vi "prueba1_520.vi"() -> ()   [LabVIEW 2011]
panel:
  out "Temperatura Mayor":dbl
  out "61-100":bool
  out "31-60":bool
  out "1-30":bool
  out "temperaturaProm":dbl
  out "temperatura":i32(slide) scale=0.0..100.0
  # "Generar la temperatura entre 1-100\nel programa se detiene cuando la\ntemperatura es mayor a 90.\nAl final debera de presentar la\ntemperatura promedio.\nDurante el programa se ejecute\ndebera de encender los led de acuerdo\nal rango.\nobtener la temperatura mayor"
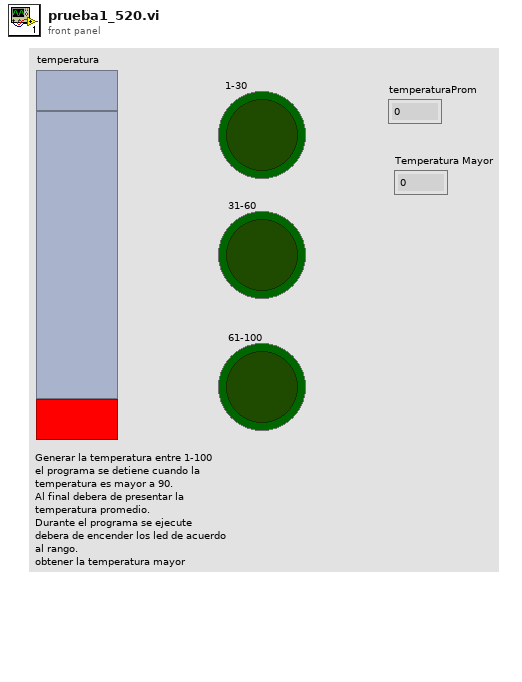
[diagram p1: front panel]
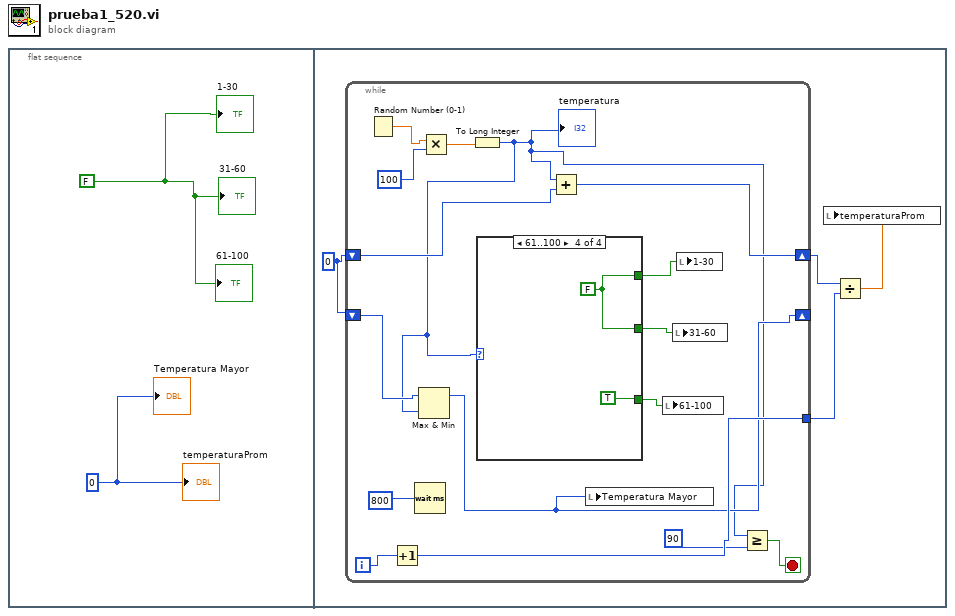
[diagram p0: block diagram]
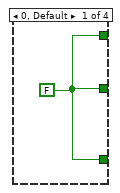
[diagram p2: hidden frame]
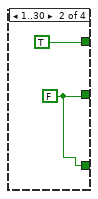
[diagram p3: hidden frame]
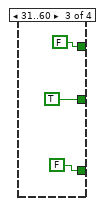
[diagram p4: hidden frame]
diagram:
  n1 = flat-sequence {
    frame #0 {
      w2 = FALSE
      w1 = 0
      "temperaturaProm" <- w1
      "1-30" <- w2
      "31-60" <- w2
      "61-100" <- w2
      "Temperatura Mayor" <- w1
    }
    frame #1 {
      w3 = 0
      n2 = while {
        shift-right: [w15] -> w6
        shift-left: w3 -> [w18]
        shift-right: [w10] -> _
        shift-left: w3 -> [w11]
        tunnel: [w16] -> w5
        i -> [w17]
        stop <- w9 stop-if-true
        n3 = Random Number (0-1)() -> (number: 0 to 1=w19:dbl)
        n4 = Increment(x=w17) -> (x+1=w16:i32)
        n5 = Wait (ms)(milliseconds to wait=800) -> ()  [unwired: 1 out]
        n6 = Multiply(x=w19, y=100) -> (x*y=w21:dbl)
        n7 = To Long Integer(number=w21) -> (32bit integer=w7:i32)
        "temperatura" <- w7
        n8 = Max & Min(x=w11, y=w7) -> (max(x,y)=w10:i32)  [unwired: 1 out]
        n9 = case shown="61..100" w7 {
          tunnel: [w23 TRUE FALSE w29] -> w14
          tunnel: [w23 w24 FALSE TRUE] -> w13
          tunnel: [w23 w24 TRUE w29] -> w12
          frame 0, Default {
            w23 = FALSE
          }
          frame 1..30 {
            w24 = FALSE
          }
          frame 31..60 {
          }
          frame 61..100 {
            w29 = FALSE
          }
        }
        n10 = Add(x=w7, y=w18) -> (x+y=w15:i32)
        n11 = local write "Temperatura Mayor"(w10) -> ()
        n12 = local write "61-100"(w13) -> ()
        n13 = local write "31-60"(w12) -> ()
        n14 = local write "1-30"(w14) -> ()
        n15 = Greater Or Equal?(x=w7, y=90) -> (x >= y?=w9:bool)
      }
      n16 = Divide(x=w6, y=w5) -> (x/y=w4:dbl)
      n17 = local write "temperaturaProm"(w4) -> ()
    }
  }
